vi "Panel.vi"(11 "2WayValveEditorPanel in":refnum<class "2WayValveEditorPanel.lvclass">) -> ()   [LabVIEW 2020, in "VolatusGUIControls.lvlib" / "2WayValveEditorPanel.lvclass"]
uses:
  2WayValveEditorPanel.lvclass
  C:/dev/lv20CE/relink/volatus-gui-controls/VolatusGUIEditorCore/ElementEditorPanel/ElementEditorPanel.lvclass
  C:/dev/lv20CE/relink/lv-oopanel/OOPanel/Panel/Panel.lvclass
  lv-oopanel/OOPanel/Panel/Basic UI State.ctl
  lv-autocomplete/AutoComplete/AutoComplete/AutoComplete.lvclass/AutoComplete.ctl
  2WayValveEditorPanel.lvclass/2WayValveEditorPanel.ctl
  lv-autocomplete/AutoComplete/Launch Autocomplete Handler.vi
  lv-autocomplete/AutoComplete/AutoComplete/AutoComplete.lvclass
  lv-oopanel/OOPanel/Panel/Panel.lvclass
  lv-oopanel/OOPanel/OOPanel.lvlib
  VolatusGUIEditorCore/ElementEditorPanel/ElementEditorPanel.lvclass
  VolatusGUIEditorCore/VolatusGUIEditorCore.lvlib
panel:
  in  "Inhibit":string caption="Channel"
  in  "Top":i32
  in  "Left":i32
  in  "Label Text Color":u32(colorbox) caption="Color"
  in  "Label Visible":bool caption="Visible"
  in  "Label":string
  in  "Energized Threshold":dbl caption="Limit" format="%.2f"
  in  "Energized":string caption="Channel"
  in  "Open FB":string caption="Channel"
  in  "Closed FB":string caption="Channel"
  in  "Output":string caption="Channel"
  # "Label"
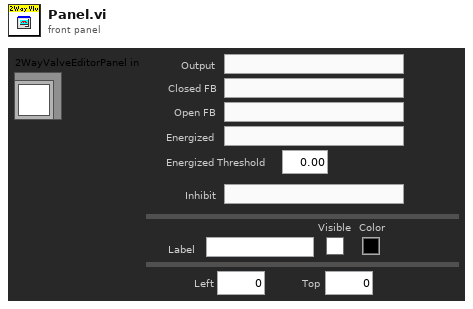
[diagram p1: front panel]
types:
  T1 = typedef "OOPanel.lvlib/Panel.lvclass/Basic UI State.ctl" = enum16{"Init", "Run", "Close"}
  T2 = typedef "VolatusGUIEditorCore.lvlib/ElementEditorPanel.lvclass/Incoming Events.ctl" = cluster{"Update Control":refnum<user-event>}
  T3 = typedef "OOPanel.lvlib/Panel.lvclass/Panel Events.ctl" = cluster{"Visbility":refnum<user-event>, "Close":refnum<user-event>}
  T4 = typedef "VolatusGUIControls.lvlib/2WayValveEditorPanel.lvclass/Props.ctl" = cluster{"JSON":T5, "Label":T6, "Position":T7}
  T5 = typedef "VolatusGUIControls.lvlib/2WayValveEditorPanel.lvclass/JSON Props.ctl" = cluster{"Output":cluster{"Channel":string}, "ClosedFB":cluster{"Channel":string}, "OpenFB":cluster{"Channel":string}, "Energized":cluster{"Channel":string, "Limit":dbl}, "Inhibit":string}
  T6 = typedef "VolatusGUIEditorCore.lvlib/Label Props.ctl" = cluster{"Text":string, "Text Color":u32, "Visible":bool}
  T7 = typedef "VolatusGUIEditorCore.lvlib/Position Props.ctl" = cluster{"Left":i32, "Top":i32}
  T8 = typedef "OOPanel.lvlib/Visibility State.ctl" = enum16{"Idle", "Closed", "Hidden", "Visible", "Subpanel", "Hidden Subpanel"}
  T9 = cluster{"Label":string, "Label Text Color":u32, "Label Visible":bool}
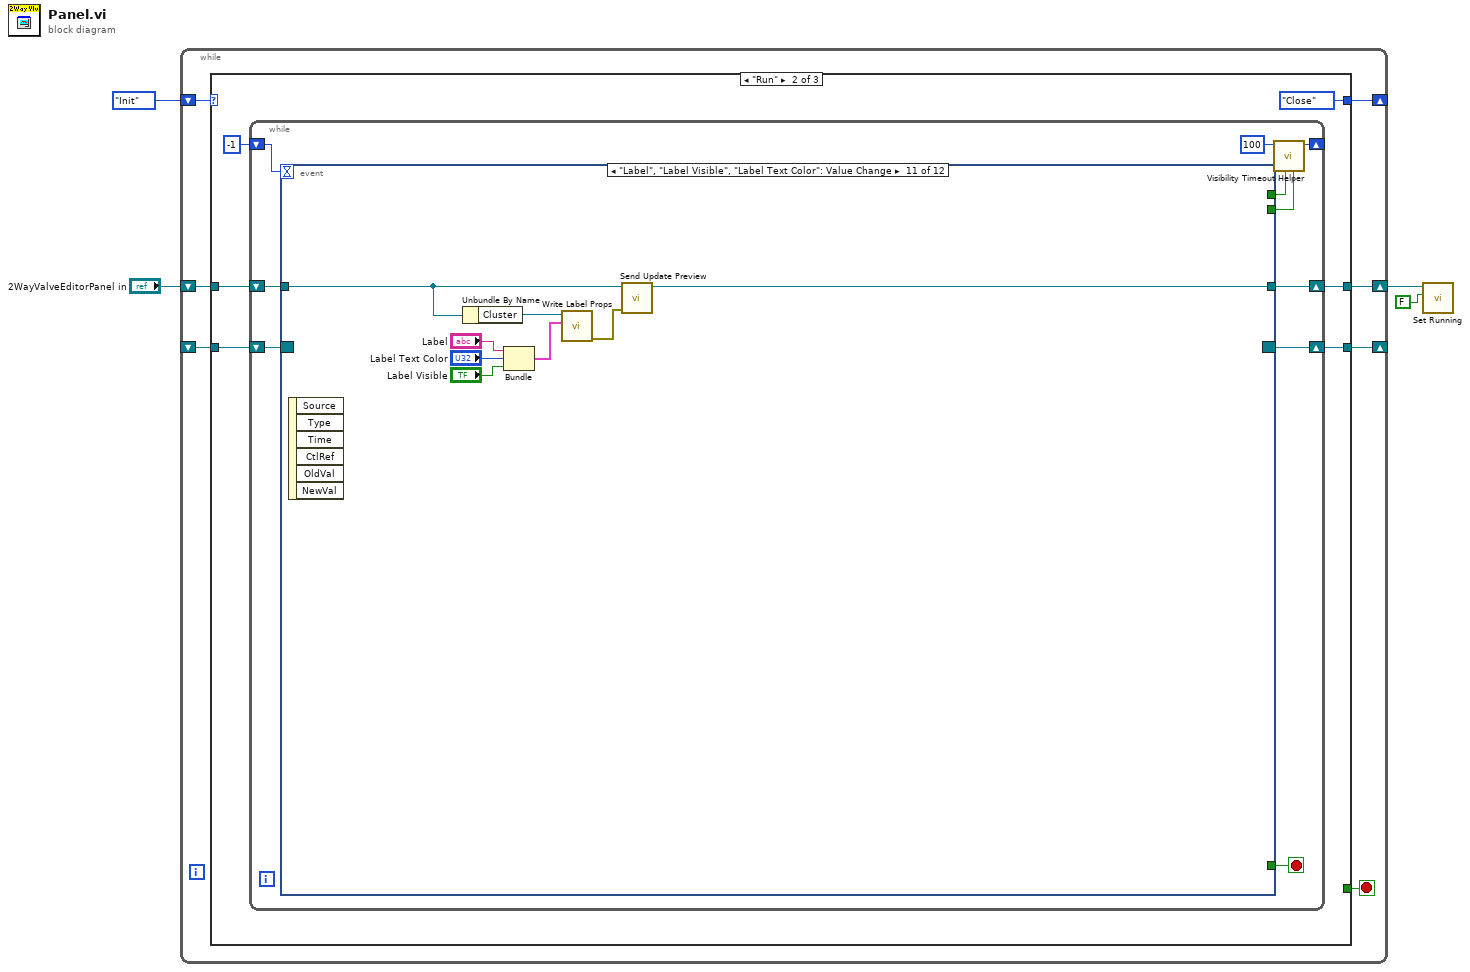
[diagram p0: block diagram]
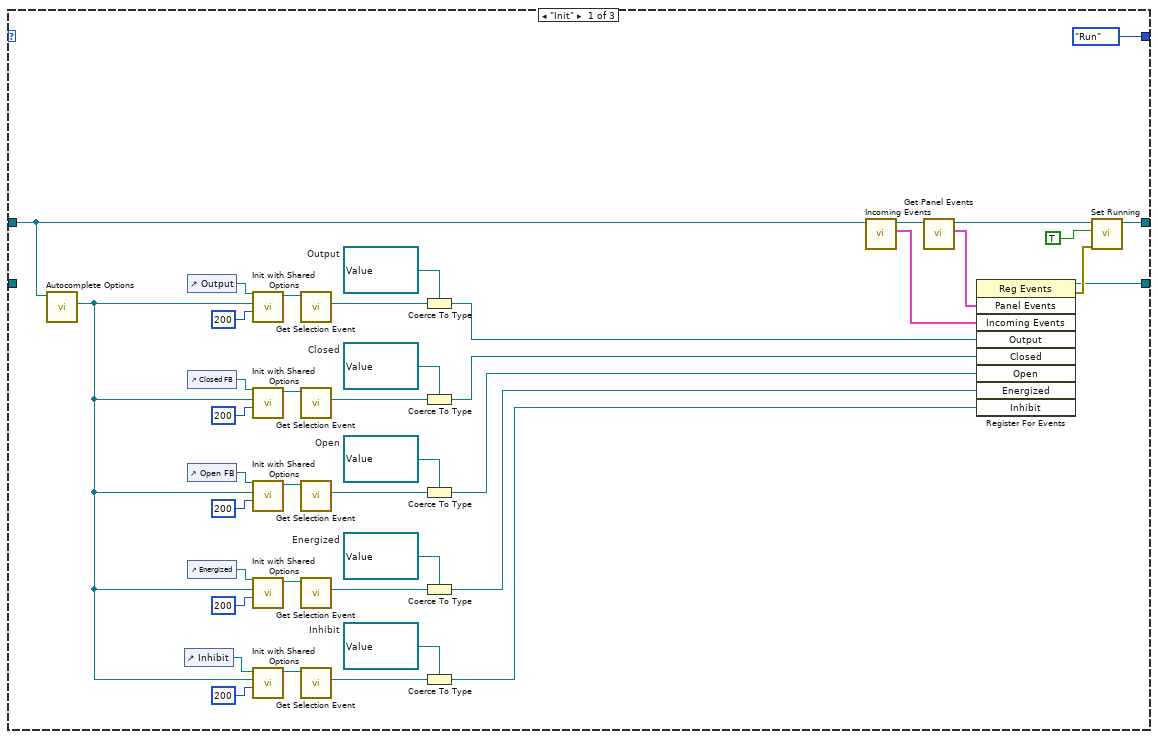
[diagram p2: hidden frame]
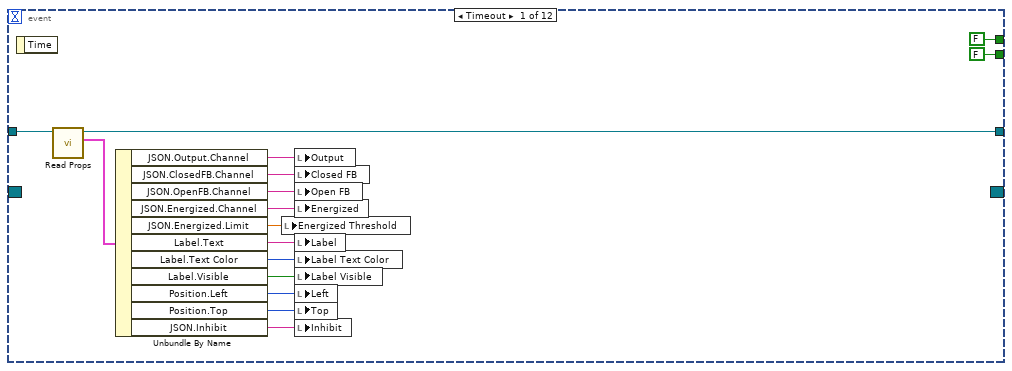
[diagram p3: hidden frame]
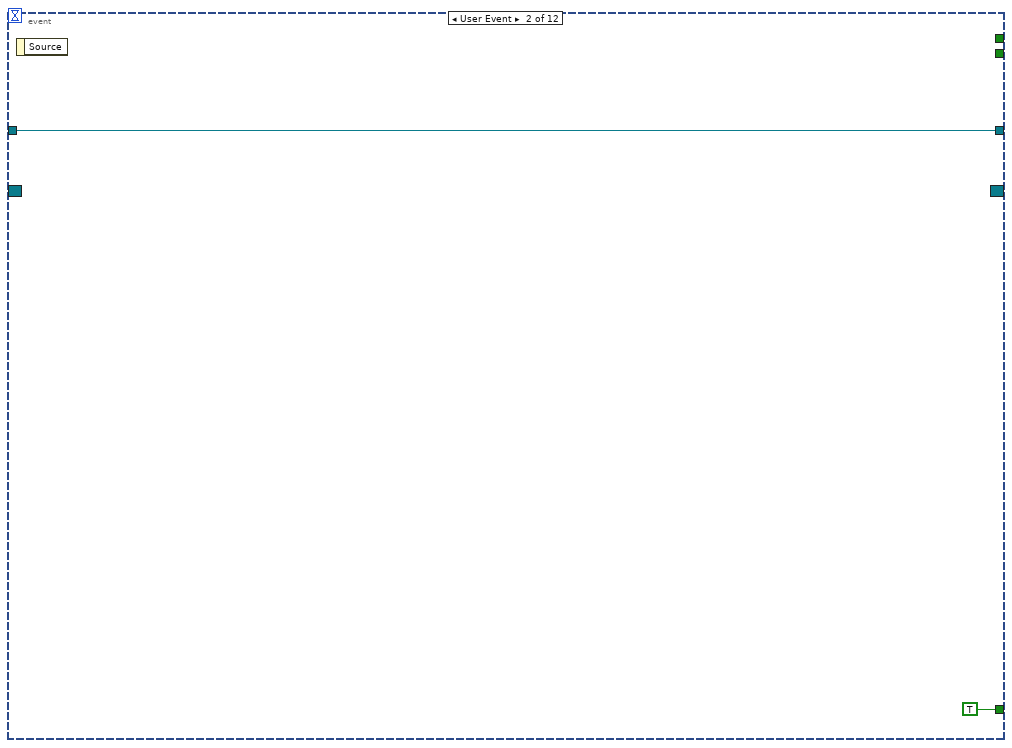
[diagram p4: hidden frame]
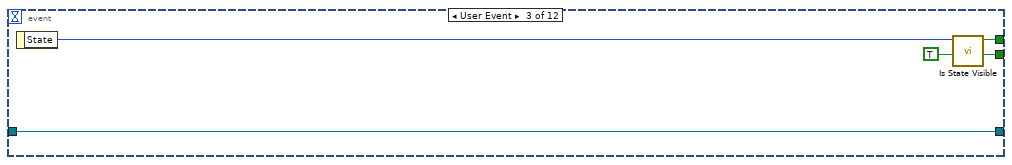
[diagram p5: hidden frame]
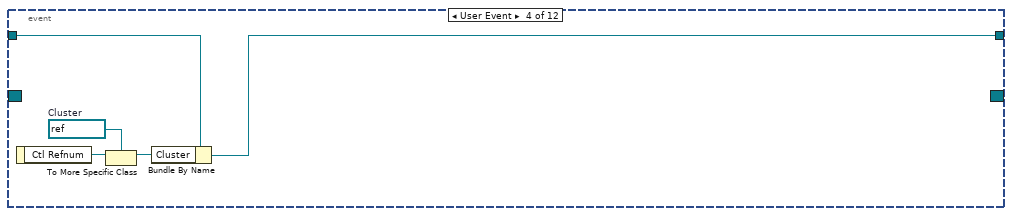
[diagram p6: hidden frame]
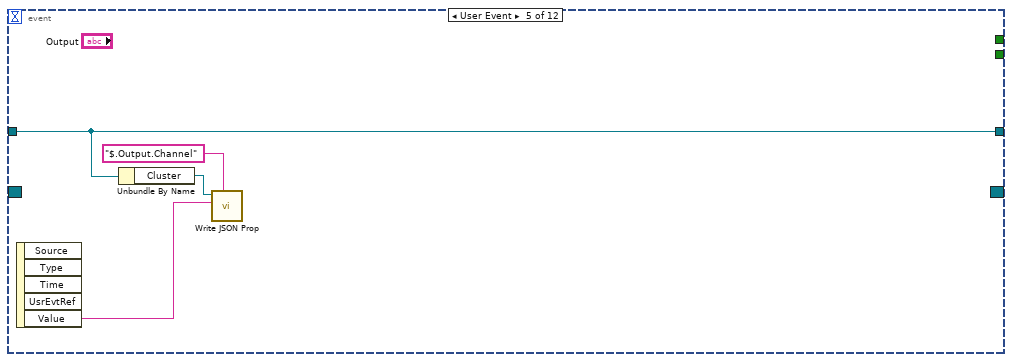
[diagram p7: hidden frame]
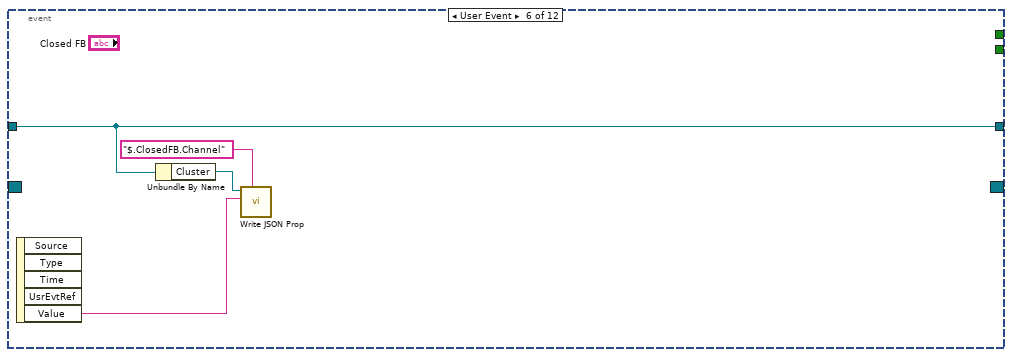
[diagram p8: hidden frame]
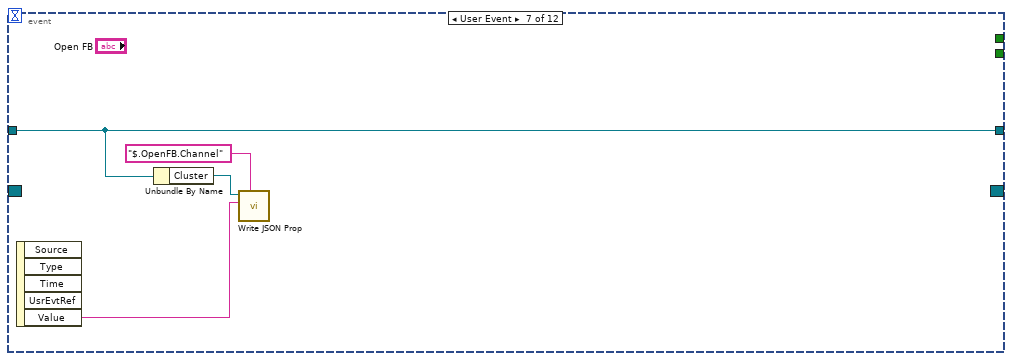
[diagram p9: hidden frame]
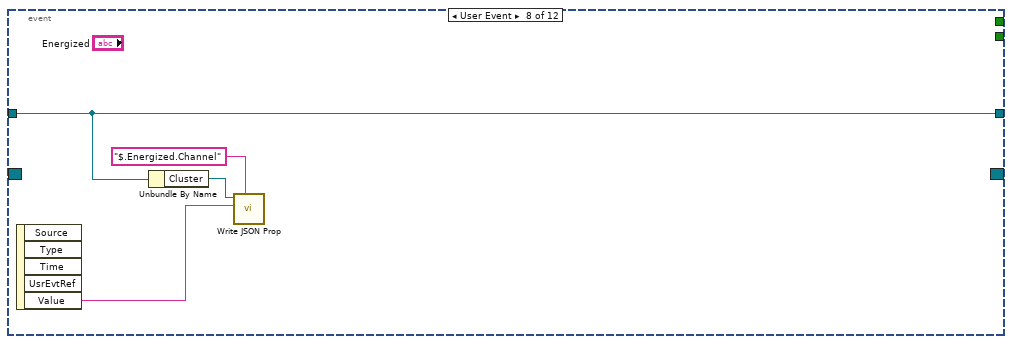
[diagram p10: hidden frame]
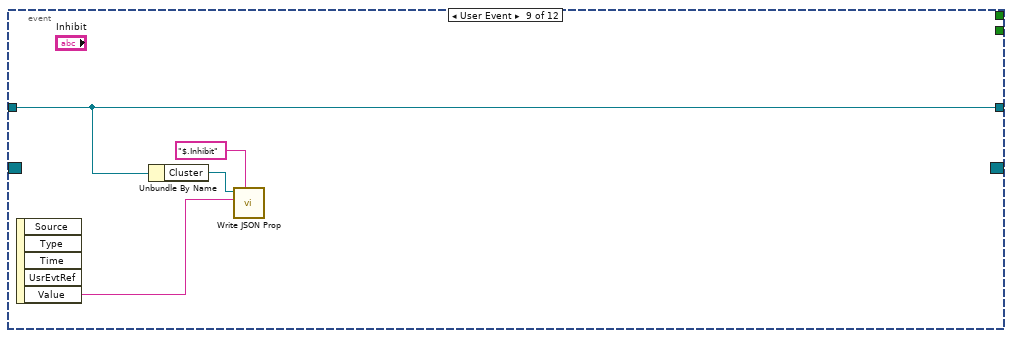
[diagram p11: hidden frame]
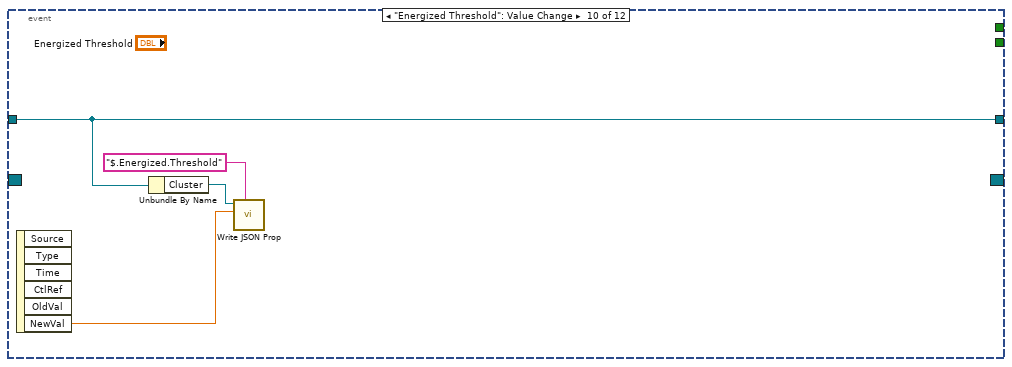
[diagram p12: hidden frame]
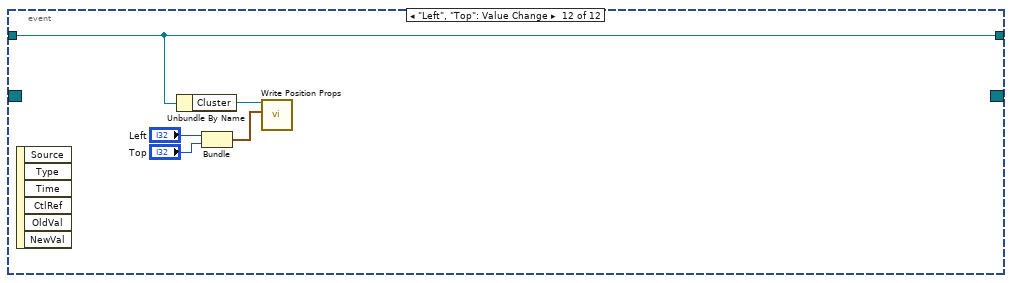
[diagram p13: hidden frame]
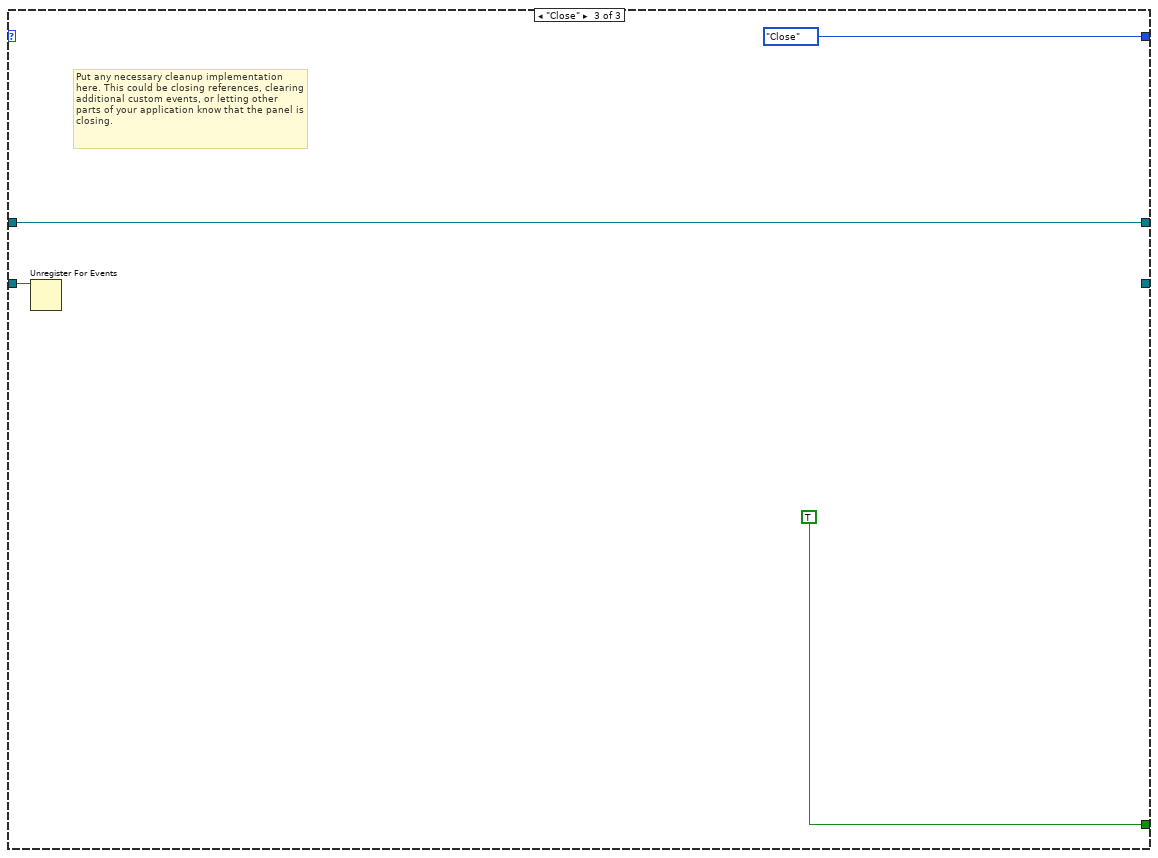
[diagram p14: hidden frame]
diagram:
  n1 = while {
    shift-right: [w10] -> _
    shift-left: _ -> [w11]
    shift-right: [w8] -> _
    shift-left: Basic_UI_State."Init" ("Basic UI State") -> [w9]
    shift-right: [w6] -> w4
    shift-left: "2WayValveEditorPanel in" -> [w5]
    stop <- w7 stop-if-true
    n2 = case shown="\"Run\"" w9 {
      tunnel: w11 -> [_ w58 w134]
      tunnel: [w49 w56 _] -> w10
      tunnel: [Basic_UI_State."Run" ("Basic UI State") Basic_UI_State."Close" ("Basic UI State") Basic_UI_State."Close" ("Basic UI State")] -> w8
      tunnel: [_ _ TRUE] -> w7
      tunnel: [w48 w53 w133] -> w6
      tunnel: w5 -> [w41 w54 w133]
      frame "Init" {
        w15 = refnum<user-event> refnum  # Inhibit
        w25 = refnum<user-event> refnum  # Energized
        w28 = refnum<user-event> refnum  # Open
        w35 = refnum<user-event> refnum  # Closed
        w39 = refnum<user-event> refnum  # Output
        n3 = call "Autocomplete Options.vi"("ElementEditorPanel in"=w41) -> ("Autocomplete Options"=w14:refnum<class "Shared Options.lvclass">)  [unwired: 10 in]
        n4 = control-ref of="Inhibit"() -> (w13:refnum<vi>)
        n5 = control-ref of="Output"() -> (w37:refnum<vi>)
        n6 = control-ref of="Closed FB"() -> (w36:refnum<vi>)
        n7 = control-ref of="Open FB"() -> (w27:refnum<vi>)
        n8 = control-ref of="Energized"() -> (w26:refnum<vi>)
        n9 = call "Init with Shared Options.vi"("Height (200)"=i16 200, "Shared Options"=w14, "Str Refnum"=w37) -> ("AutoComplete out"=w43:refnum<class "AutoComplete.lvclass">)  [unwired: 7 in, 1 out]
        n10 = call "Init with Shared Options.vi"("Height (200)"=i16 200, "Shared Options"=w14, "Str Refnum"=w36) -> ("AutoComplete out"=w32:refnum<class "AutoComplete.lvclass">)  [unwired: 7 in, 1 out]
        n11 = call "Init with Shared Options.vi"("Height (200)"=i16 200, "Shared Options"=w14, "Str Refnum"=w27) -> ("AutoComplete out"=w31:refnum<class "AutoComplete.lvclass">)  [unwired: 7 in, 1 out]
        n12 = call "Init with Shared Options.vi"("Height (200)"=i16 200, "Shared Options"=w14, "Str Refnum"=w26) -> ("AutoComplete out"=w22:refnum<class "AutoComplete.lvclass">)  [unwired: 7 in, 1 out]
        n13 = call "Init with Shared Options.vi"("Height (200)"=i16 200, "Shared Options"=w14, "Str Refnum"=w13) -> ("AutoComplete out"=w18:refnum<class "AutoComplete.lvclass">)  [unwired: 7 in, 1 out]
        n14 = call "Get Selection Event.vi"("AutoComplete in"=w43) -> ("Selection Event"=w40:refnum<user-event>)  [unwired: 9 in, 1 out]
        n15 = call "Get Selection Event.vi"("AutoComplete in"=w32) -> ("Selection Event"=w34:refnum<user-event>)  [unwired: 9 in, 1 out]
        n16 = call "Get Selection Event.vi"("AutoComplete in"=w31) -> ("Selection Event"=w29:refnum<user-event>)  [unwired: 9 in, 1 out]
        n17 = call "Get Selection Event.vi"("AutoComplete in"=w22) -> ("Selection Event"=w24:refnum<user-event>)  [unwired: 9 in, 1 out]
        n18 = call "Get Selection Event.vi"("AutoComplete in"=w18) -> ("Selection Event"=w16:refnum<user-event>)  [unwired: 9 in, 1 out]
        n19 = Coerce To Type(0:w40, 1:w39) -> (2:w38:refnum<user-event>)
        n20 = Coerce To Type(0:w34, 1:w35) -> (2:w21:refnum<user-event>)
        n21 = Coerce To Type(0:w29, 1:w28) -> (2:w20:refnum<user-event>)
        n22 = Coerce To Type(0:w24, 1:w25) -> (2:w19:refnum<user-event>)
        n23 = Coerce To Type(0:w16, 1:w15) -> (2:w12:refnum<user-event>)
        n24 = call "Incoming Events.vi"("ElementEditorPanel in"=w41) -> ("Incoming Events"=w44:T2, "ElementEditorPanel out"=w45:refnum<class "2WayValveEditorPanel.lvclass">)  [unwired: 9 in]
        n25 = call "Get Panel Events.vi"("Panel in"=w45) -> ("Panel Events"=w46:T3, "Panel out"=w47:refnum<class "2WayValveEditorPanel.lvclass">)  [unwired: 8 in, 1 out]
        n26 = register-events(w46, w44, w38, w21, w20, w19, w12) -> (reference out=w49:refnum<event-registration>, error out=w51:errorcluster)  [unwired: 2 in]
        n27 = call "Set Running.vi"("error in (no error)"=w51, "Running"=TRUE, "Panel in"=w47) -> ("Panel out"=w48:refnum<class "2WayValveEditorPanel.lvclass">)  [unwired: 7 in, 1 out]
      }
      frame "Run" {
        n28 = while {
          shift-right: [w64] -> w56
          shift-left: w58 -> [w65]
          shift-right: [w67] -> _
          shift-left: -1 ("Timeout") -> [w66]
          shift-right: [w59] -> w53
          shift-left: w54 -> [w60]
          stop <- w61 stop-if-true
          n29 = event shown="[10] \"Label\", \"Label Visible\", \"Label Text Color\": Value Change" {
            selector: w65 -> [_ _ _ _ _ _ _ _ _ _ _ _]
            dyn-events: [_ _ _ _ _ _ _ _ _ _ _ _] -> w64
            timeout: w66 -> [_ _ _ _ _ _ _ _ _ _ _ _]
            tunnel: [FALSE _ w89 _ _ _ _ _ _ _ _ _] -> w63
            tunnel: [FALSE _ TRUE _ _ _ _ _ _ _ _ _] -> w62
            tunnel: [_ TRUE _ _ _ _ _ _ _ _ _ _] -> w61
            tunnel: w60 -> [w81 w85 w87 w95 w97 w101 w105 w109 w113 w117 w127 w129]
            tunnel: [w82 w85 w87 w92 w97 w101 w105 w109 w113 w117 w121 w129] -> w59
            event Timeout {
              n30 = event-data() -> ()  [unwired: 1 in, 1 out]
              n31 = call "Read Props.vi"("2WayValveEditorPanel in"=w81) -> ("Props"=w80:T4, "2WayValveEditorPanel out"=w82:refnum<class "2WayValveEditorPanel.lvclass">)  [unwired: 8 in, 1 out]
              n32 = Unbundle By Name(w80) -> ("JSON.Output.Channel"=w79:string, "JSON.ClosedFB.Channel"=w70:string, "JSON.OpenFB.Channel"=w71:string, "JSON.Energized.Channel"=w72:string, "JSON.Energized.Limit"=w73:dbl, "Label.Text"=w74:string, "Label.Text Color"=w75:u32, "Label.Visible"=w76:bool, "Position.Left"=w77:i32, "Position.Top"=w78:i32, "JSON.Inhibit"=w69:string)
              n33 = local write "Energized Threshold"(w73) -> ()
              n34 = local write "Output"(w79) -> ()
              n35 = local write "Closed FB"(w70) -> ()
              n36 = local write "Open FB"(w71) -> ()
              n37 = local write "Energized"(w72) -> ()
              n38 = local write "Label"(w74) -> ()
              n39 = local write "Label Text Color"(w75) -> ()
              n40 = local write "Label Visible"(w76) -> ()
              n41 = local write "Left"(w77) -> ()
              n42 = local write "Top"(w78) -> ()
              n43 = local write "Inhibit"(w69) -> ()
            }
            event User Event {
              n44 = event-data() -> ()  [unwired: 1 in, 1 out]
            }
            event User Event {
              n45 = event-data() -> ("State"=w90:T8)  [unwired: 1 in]
              n46 = call "Is State Visible.vi"("Visibility"=w90) -> ("Visible"=w89:bool)  [unwired: 10 in]
            }
            event User Event {
              w93 = refnum<vi> refnum  # Cluster
              n47 = event-data() -> ("Ctl Refnum"=w94:refnum<vi>)  [unwired: 1 in]
              n48 = To More Specific Class(target class=w93, reference=w94) -> (specific class reference=w91:refnum<vi>)  [unwired: 1 in, 1 out]
              n49 = Bundle By Name(cluster=w95, "Cluster"=w91) -> (w92:refnum<class "2WayValveEditorPanel.lvclass">)
            }
            event User Event {
              n50 = event-data() -> ("Value"=w96:string)  [unwired: 1 in, 4 out]
              n51 = Unbundle By Name(w97) -> ("Cluster"=w99:refnum<vi>)
              n52 = call "Write JSON Prop.vi"("JSON Path"="$.Output.Channel" ("$Path or Item Name"), "Value"=w96, "Ctl Refnum in"=w99) -> ()  [unwired: 7 in, 2 out]
            }
            event User Event {
              n53 = event-data() -> ("Value"=w100:string)  [unwired: 1 in, 4 out]
              n54 = Unbundle By Name(w101) -> ("Cluster"=w103:refnum<vi>)
              n55 = call "Write JSON Prop.vi"("JSON Path"="$.ClosedFB.Channel" ("$Path or Item Name"), "Value"=w100, "Ctl Refnum in"=w103) -> ()  [unwired: 7 in, 2 out]
            }
            event User Event {
              n56 = event-data() -> ("Value"=w104:string)  [unwired: 1 in, 4 out]
              n57 = Unbundle By Name(w105) -> ("Cluster"=w107:refnum<vi>)
              n58 = call "Write JSON Prop.vi"("JSON Path"="$.OpenFB.Channel" ("$Path or Item Name"), "Value"=w104, "Ctl Refnum in"=w107) -> ()  [unwired: 7 in, 2 out]
            }
            event User Event {
              n59 = event-data() -> ("Value"=w108:string)  [unwired: 1 in, 4 out]
              n60 = Unbundle By Name(w109) -> ("Cluster"=w111:refnum<vi>)
              n61 = call "Write JSON Prop.vi"("JSON Path"="$.Energized.Channel" ("$Path or Item Name"), "Value"=w108, "Ctl Refnum in"=w111) -> ()  [unwired: 7 in, 2 out]
            }
            event User Event {
              n62 = event-data() -> ("Value"=w112:string)  [unwired: 1 in, 4 out]
              n63 = Unbundle By Name(w113) -> ("Cluster"=w115:refnum<vi>)
              n64 = call "Write JSON Prop.vi"("JSON Path"="$.Inhibit" ("$Path or Item Name"), "Value"=w112, "Ctl Refnum in"=w115) -> ()  [unwired: 7 in, 2 out]
            }
            event "Energized Threshold": Value Change {
              n65 = event-data() -> ("NewVal"=w116:dbl)  [unwired: 1 in, 5 out]
              n66 = Unbundle By Name(w117) -> ("Cluster"=w119:refnum<vi>)
              n67 = call "Write JSON Prop.vi"("JSON Path"="$.Energized.Threshold" ("$Path or Item Name"), "Value"=w116, "Ctl Refnum in"=w119) -> ()  [unwired: 7 in, 2 out]
            }
            event "Label", "Label Visible", "Label Text Color": Value Change {
              n68 = event-data() -> ()  [unwired: 1 in, 6 out]
              n69 = Unbundle By Name(w127) -> ("Cluster"=w126:refnum<vi>)
              n70 = Bundle("Label"="Label", "Label Text Color"="Label Text Color", "Label Visible"="Label Visible") -> (w122:T9)  [unwired: 1 in]
              n71 = call "Write Label Props.vi"("Label Props"=w122, "Ctl Refnum in"=w126) -> ("error out"=w120:errorcluster)  [unwired: 8 in, 1 out]
              n72 = call "Send Update Preview.vi"("error in (no error)"=w120, "ElementEditorPanel in"=w127) -> ("ElementEditorPanel out"=w121:refnum<class "2WayValveEditorPanel.lvclass">)  [unwired: 8 in, 1 out]
            }
            event "Left", "Top": Value Change {
              n73 = event-data() -> ()  [unwired: 1 in, 6 out]
              n74 = Unbundle By Name(w129) -> ("Cluster"=w128:refnum<vi>)
              n75 = Bundle("Left"="Left", "Top"="Top") -> (w130:cluster{"Left":i32, "Top":i32})  [unwired: 1 in]
              n76 = call "Write Position Props.vi"("Position Props"=w130, "Ctl Refnum in"=w128) -> ()  [unwired: 8 in, 2 out]
            }
          }
          n77 = call "Visibility Timeout Helper.vi"("Update?"=w62, "Use Timeout?"=w63, "Visible Timeout mS"=100) -> ("Timeout"=w67:i32)  [unwired: 8 in]
        }
      }
      frame "Close" {
        # "Put any necessary cleanup implementation here. This could be closing references, clearing additional custom events, or letting other parts of your application know that the panel is closing."
        n78 = Unregister For Events(event registration refnum=w134) -> ()  [unwired: 1 in, 1 out]
      }
    }
  }
  n79 = call "Set Running.vi"("Running"=FALSE, "Panel in"=w4) -> ()  [unwired: 8 in, 2 out]
